vi "DB_Fast Cash.vi"() -> ()   [LabVIEW 2013, in "ConfigDBLib.lvlib"]
uses:
  ConfigDBLib.lvlib
panel:
  in  "Total Balance":dbl
  in  "Account Number":dbl
  out "error out":errorcluster
  in  "error in (no error)":errorcluster
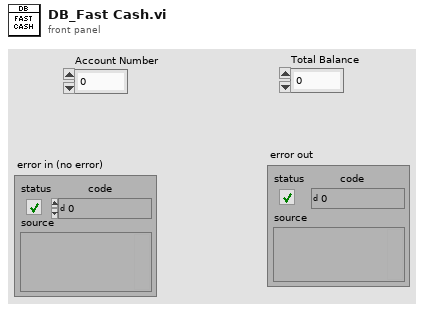
[diagram p1: front panel]
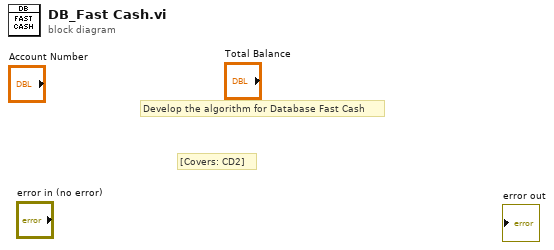
[diagram p0: block diagram]
diagram:
  # "[Covers: CD2]"
  # "Develop the algorithm for Database Fast Cash"
